vi "FGVScanClocks.vi"(5 "Enum":T2, 6 "error in":errorcluster, 9 "scanClocksInput":T1) -> (0 "error out":errorcluster, 3 "scanClocksOutput":T1)   [LabVIEW 2016]
uses:
  controls/Enum.ctl
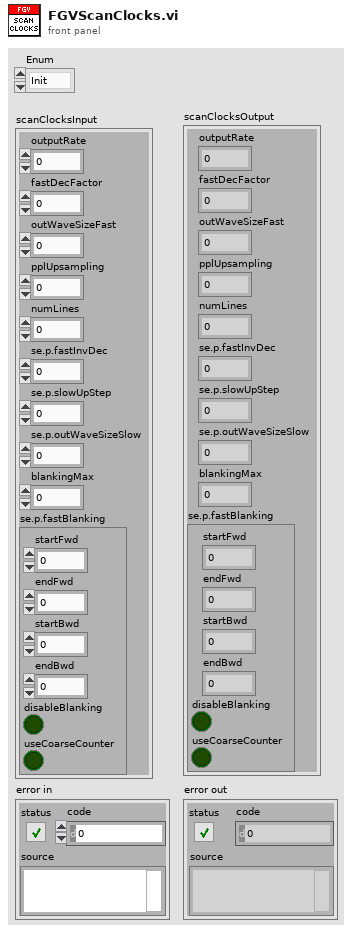
[diagram p1: front panel]
types:
  T1 = cluster{"outputRate":u16, "fastDecFactor":u16, "outWaveSizeFast":u16, "pplUpsampling":u16, "numLines":u16, "se.p.fastInvDec":fxp<+,22,0>, "se.p.slowUpStep":fxp<+,28,0>, "se.p.outWaveSizeSlow":u16, "blankingMax":u32, "se.p.fastBlanking":cluster{"startFwd":u32, "endFwd":u32, "startBwd":u32, "endBwd":u32, "disableBlanking":bool, "useCoarseCounter":bool}}
  T2 = typedef "Enum.ctl" = enum16{"Init", "Read", "Write"}
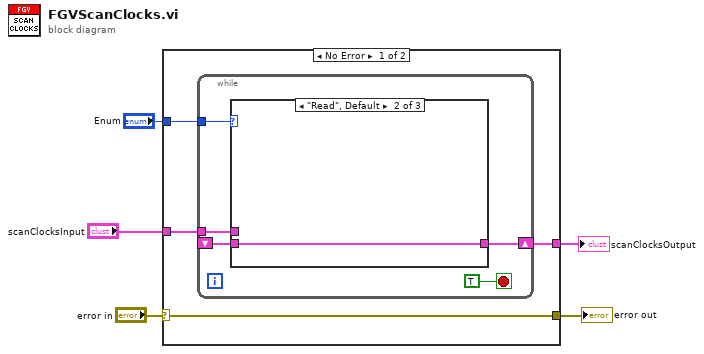
[diagram p0: block diagram]
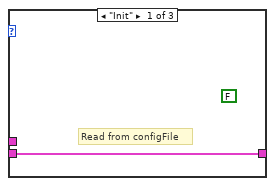
[diagram p2: hidden frame]
diagram:
  n1 = case shown="No Error" "error in" {
    selector: "error in" -> [w8 w19]
    tunnel: "Enum" -> [w9 _]
    tunnel: [w8 w19] -> w4
    tunnel: "scanClocksInput" -> [w7 w18]
    tunnel: [w6 w18] -> w1
    frame No Error {
      n2 = while {
        tunnel: w9 -> [w13]
        tunnel: w7 -> [w12]
        shift-right: [w11] -> w6
        shift-left: _ -> [w10]
        stop <- TRUE stop-if-true
        n3 = case shown="\"Read\", Default" w13 {
          tunnel: w12 -> [_ _ w17]
          tunnel: [w15 w16 w17] -> w11
          tunnel: w10 -> [w15 w16 _]
          frame "Init" {
            (unwired) FALSE
            # "Read from configFile"
          }
          frame "Read", Default {
          }
          frame "Write" {
          }
        }
      }
    }
    frame Error {
    }
  }
  "error out" <- w4
  "scanClocksOutput" <- w1
